vi "Read Snippet.vi"(8 "error in (no error)":errorcluster, 11 "VI Snippet (.png)":path) -> (0 "error out":errorcluster, 3 "Snippet":T1)   [LabVIEW 2022 SP3, in "VI-Snippet.lvlib"]
doc: "Reads a VI Snippet image and extracts the embedded VI."
uses:
  VI-Snippet.lvlib
  Snippet.ctl
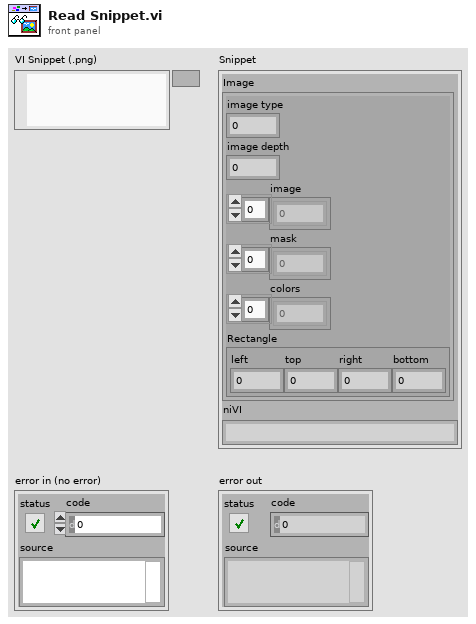
[diagram p1: front panel]
types:
  T1 = typedef "VI-Snippet.lvlib/Snippet.ctl" = cluster{"Image":cluster{"image type":i32, "image depth":i32, "image":u8[], "mask":u8[], "colors":u32[], "Rectangle":cluster{"left":i16, "top":i16, "right":i16, "bottom":i16}}, "niVI":string}
  T2 = typedef "imagedata.ctl" = cluster{"image type":i32, "image depth":i32, "image":u8[], "mask":u8[], "colors":u32[], "Rectangle":cluster{"left":i16, "top":i16, "right":i16, "bottom":i16}}
  T3 = cluster{"Length":i32, "Type":string, "Data":string, "CRC":u32}[]
  T4 = cluster{"Length":i32, "Type":string, "Data":string, "CRC":u32}
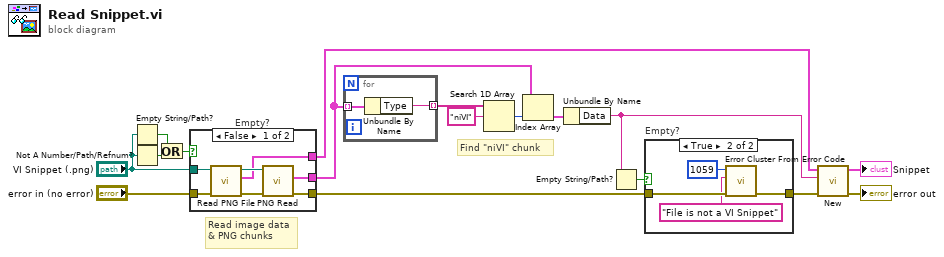
[diagram p0: block diagram]
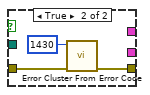
[diagram p2: hidden frame]
diagram:
  # "Read image data\n& PNG chunks"
  # "Find \"niVI\" chunk"
  n1 = Empty String/Path?(string/path="VI Snippet (.png)") -> (empty?=w9:bool)
  n2 = Not A Number/Path/Refnum?(number/path/refnum="VI Snippet (.png)") -> (NaN/Path/Refnum?=w8:bool)
  n3 = Or(x=w9, y=w8) -> (x .or. y?=w7:bool)
  n4 = case "Empty?" shown="False" w7 {
    tunnel: "error in (no error)" -> [w24 w27]
    tunnel: "VI Snippet (.png)" -> [w23 _]
    tunnel: [w20 w26] -> w12
    tunnel: [w19 _] -> w10
    tunnel: [w18 _] -> w3
    frame False {
      n5 = call <vilib>:"Read PNG File.vi"("error in (no error)"=w24, "path to PNG file"=w23) -> ("error out"=w21:errorcluster, "image data"=w18:T2, "path"=w22:path)  [unwired: 7 in]
      n6 = call "PNG Read.vi"("error in (no error)"=w21, "Image Path (*.png)"=w22) -> ("error out"=w20:errorcluster, "Chunks"=w19:T3)  [unwired: 7 in, 1 out]
    }
    frame True {
      n7 = call <vilib>:"Error Cluster From Error Code.vi"("error in (no error)"=w27, "error code (0)"=1430) -> ("error out"=w26:errorcluster)  [unwired: 7 in]
    }
  }
  n8 = for {
    tunnel: w10 -> [w29] mode=indexing
    tunnel: [w28] -> w16 mode=indexing
    n9 = Unbundle By Name(w29) -> ("Type"=w28:string)
  }
  n10 = Search 1D Array(1D array=w16, element="niVI" ("Type")) -> (index of element=w14:i32)  [unwired: 1 in]
  n11 = Index Array(array=w10, index=w14) -> (element=w13:T4)
  n12 = Unbundle By Name(w13) -> ("Data"=w2:string)
  n13 = Empty String/Path?(string/path=w2) -> (empty?=w11:bool)
  n14 = case "Empty?" shown="True" w11 {
    tunnel: w12 -> [w30 w34]
    tunnel: [w30 w33] -> w5
    frame False {
    }
    frame True {
      n15 = call <vilib>:"Error Cluster From Error Code.vi"("error in (no error)"=w34, "error message (\"\")"="File is not a VI Snippet" ("error message (\"\")"), "error code (0)"=1059 ("code")) -> ("error out"=w33:errorcluster)  [unwired: 6 in]
    }
  }
  n16 = call "New.vi"("error in (no error)"=w5, "niVI"=w2, "Image"=w3) -> ("error out"=→"error out":errorcluster, "VI Snippet out"=→"Snippet":T1)  [unwired: 7 in]
